vi "Read Parent Menu.vi"(8 "error in (no error)":errorcluster, 11 "NIVS_CD Template in":refnum<class "NIVS_CD Template.lvclass">) -> (0 "error out":errorcluster, 2 "Parent Menu":string, 3 "NIVS_CD Template out":refnum<class "NIVS_CD Template.lvclass">)   [LabVIEW 2019, in "NIVS_CD Template.lvclass"]
uses:
  NIVS_CD Template.lvclass
  NIVS_CD Template.lvclass/NIVS_CD Template.ctl
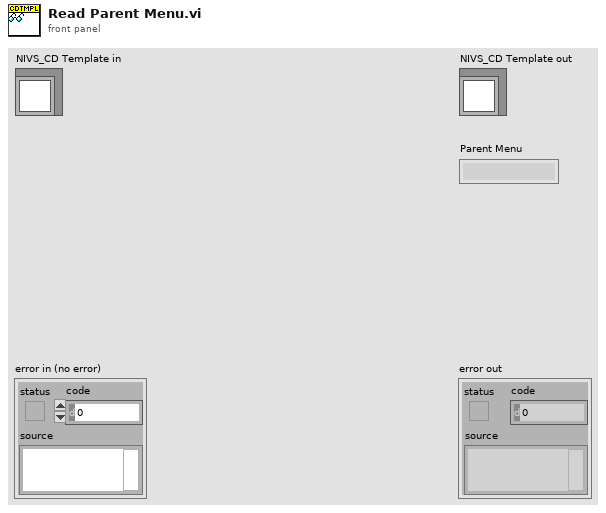
[diagram p1: front panel]
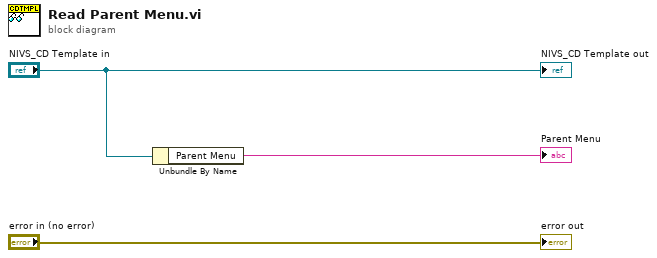
[diagram p0: block diagram]
diagram:
  n1 = Unbundle By Name("NIVS_CD Template in") -> ("Parent Menu"=→"Parent Menu":string)
  "error out" <- "error in (no error)"
  "NIVS_CD Template out" <- "NIVS_CD Template in"
